vi "Convert PGN + SA to J1939 ID.vi"(0 "PGN":u32, 7 "Source Address":u8) -> (8 "ARB ID":u32)   [LabVIEW 2015, in "J1939 Addon Shared.lvlib" / "J1939 Utilities.lvlib"]
uses:
  J1939 Utilities.lvlib
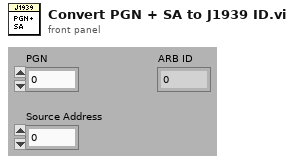
[diagram p1: front panel]
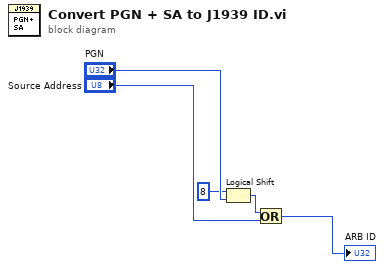
[diagram p0: block diagram]
diagram:
  n1 = Logical Shift(y=u32 8 ("x"), x="PGN") -> (x << y=w1:u32)
  n2 = Or(x=w1, y="Source Address") -> (x .or. y?=→"ARB ID":u32)
